vi "IV.vi"(2 "Run uninterrupted?":bool, 3 "Device Category IN:":string(combo)="Mini" caption="Device Category:", 4 "Batch No. IN:":string caption="Batch No.:", 5 "Sensor Serial No. IN:":string caption="Sensor Serial No.:", 6 "DB Serial No. IN:":string caption="DB Serial No.:") -> (0 "Done!":bool)   [LabVIEW 2019]
doc: "Performs IV measurements according to ATLAS ITk Quality Control Specifications."
uses:
  general_VIs/globals/QC_MeasurementSetup.vi
  general_VIs/globals/QC_RunInformation.vi
  InstrControl/InstrumentSetup.vi
  InstrControl/Switching/Switching.lvclass
  InstrControl/SupplyControl/SupplyControl.lvclass
  InstrControl/ArduinoControl/ArduinoControl.lvclass
  <vilib>/Analysis/NI_AALBase.lvlib
  InstrControl/InstrControl.lvclass
panel:
  out "Measurement Configuration Tab":enum32{"IV Setup", "IV Scan"}(tab)
  in  "V_breakdown limit [V]":dbl=-500.0
  in  "Set current limit?":bool
  in  "Current Limit [µA]":dbl=1000.0 min=0.0001 format="%.3f"
  in  "Measurement Configurations":bool
  in  "hold steps IN":i32=6 caption="hold steps"
  in  "Initial volts [V] IN":dbl caption="Initial volts [V]"
  in  "Final volts [V] IN":dbl=-700.0 caption="Final volts [V]"
  in  "step [V] IN":dbl=10.0 caption="step [V]" format="%.1f"
  in  "step interval [s] IN":i32=10 caption="step interval [s]"
  in  "Continue":bool
  in  "Quit":bool
  out "hold steps":i32=6
  out "RH":dbl[](array[numeric]) caption="RH [%]" format="%#.2f"
  out "Temp.":dbl[](array[numeric]) caption="Temp. [°C]" format="%#.2f"
  out "Current":dbl[](array[numeric]) caption="Current [nA]"
  out "Volts":dbl[](array[numeric]) caption="Volts [V]"
  out "step interval [s]":i32=10
  out "step [V]":dbl=10.0 format="%.1f"
  out "Final volts [V]":dbl=-700.0 format="%.1f"
  out "Initial volts [V]":dbl format="%.1f"
  out "Igraph":cluster{dbl[], dbl[]}(graph)
  in  "Scales":T1(ring)
  in  "Iscale":enum16{"nanoAmps", "microAmps", "milliAmps"}(ring)
  out "positive ramp?":bool
  out "DUT Description/Hardware Tab":enum32{"IV Setup", "IV Scan"}(tab)
  in  "Switching":string(combo)="LXIPXI Switching"
  in  "Hardware Configurations":bool
  in  "User:":string(combo)="Xavi"
  in  "IV Supply":string(combo)="Keithley 2410"
  in  "Temperature":enum16{"Read Arduino", "Enter manually"}(ring)
  in  "Manufacturer:":string(combo)="Hamamatsu"
  in  "abort":bool
  out "Device Category:":string
  out "DB Serial No.:":string
  out "Current Volts:":dbl format="%.2f"
  in  "quit (no save)":bool
  in  "Quit & Save":bool
  out "Bias On/Off:":bool
  out "STATUS 1":string
  out "Initiated:":string
  out "Sensor No.:":string
  out "No of steps":u32
  out "Current reading No.":u32
  out "Last reading at:":string
  # "University of\nCambridge"
  # "Strip Sensor QC: IV"
  # "Vertical Scale:"
  # "Measurement Configuration"
  # "IV Scan parameters:"
  # "Last 5 readings:"
  # "n-4"
  # "n-3"
  # "n-2"
  # "n-1"
  # "n"
  # "DUT Description"
  # "Hardware"
  # "DUT & Test Description:"
  # "Current status:"
  # "Rdg No:"
  # "out of"
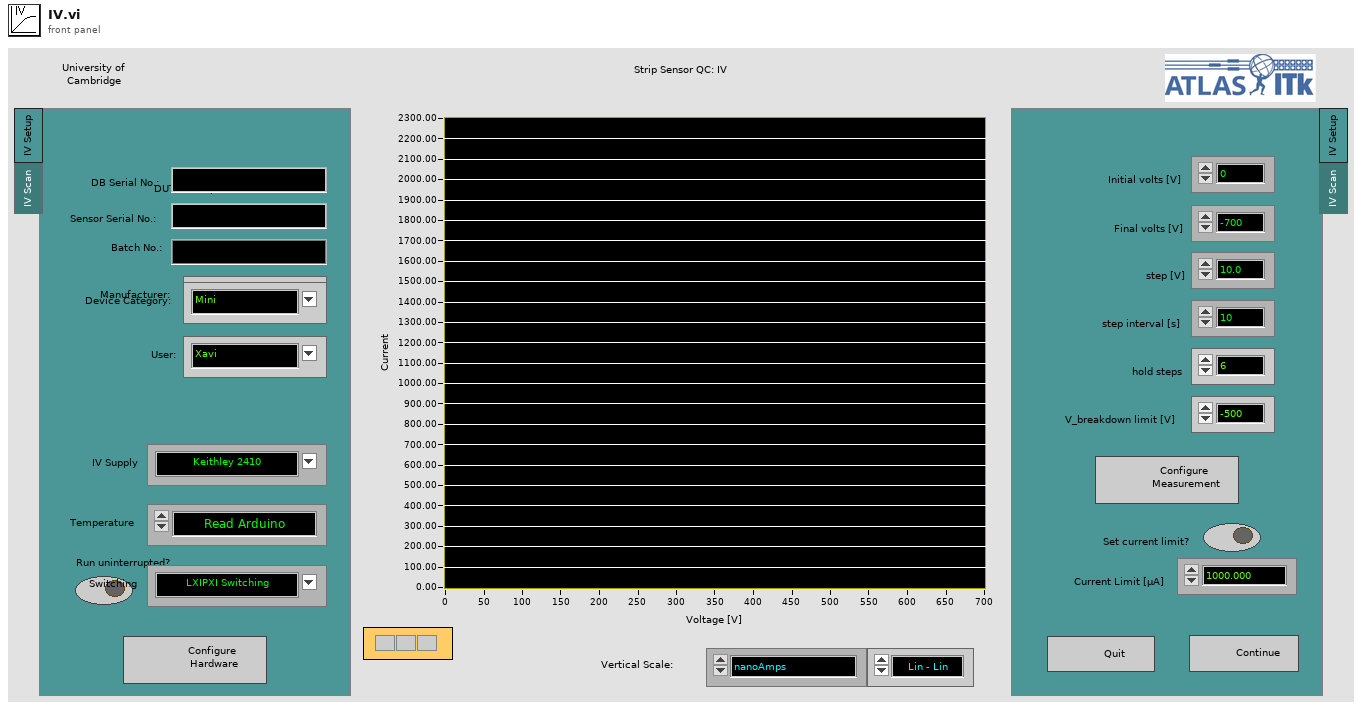
[diagram p1: front panel]
types:
  T1 = enum16{"Lin - Lin", "Log - Lin", "Lin - Log", "Log - log"}
  T2 = enum16{"Supply", "LCR", "Multimeter", "Switching"}
  T3 = enum16{"Reset", "Read Array", "Read Element", "Write Element", "Write Array", "Add Element", "Add Array"}
  T4 = enum16{"Reset", "Ground", "Striptest Bias", "Striptest SMU", "Striptest LCR", "IV", "CV", "Interstrip Cap", "Interstrip Res"}
  T5 = enum32{"IV", "CV", "Stability", "Striptest", "Cis", "Ris", "PTP"}
  T6 = cluster{"Supply":refnum<class "SupplyControl.lvclass">, "Initial Voltage [V]":dbl, "Final Voltage [V]":dbl, "Step Size [V]":dbl, "Step Interval [s]":i32, "Number Of Steps":u32, "Ramp down steps [V]":dbl, "Ramp down Interval [s]":i32, "hold steps":i32, "Set Current Limit?":bool, "Current Limit [µA]":dbl, "Temperature Readout":enum16{"Read Arduino", "Enter manually"}, "Arduino":refnum<class "ArduinoControl.lvclass">, "Supply Name":string, "V_breakdown Limit [V]":dbl, "Switching":refnum<class "Switching.lvclass">, "Matrix used?":bool, "Matrix X Channels":cluster{"Bias Supply / SMU LO":i32, "Bias Supply / SMU HI":i32, "CV Box LO":i32, "CV Box HI":i32, "CV Box LO IN":i32, "CV Box HI IN":i32, "Volt meter LO":i32, "Volt meter HI":i32, "Mux1 C1":i32, "Mux1 C2":i32, "Mux2 C1":i32, "Mux2 C2":i32}}
  T7 = cluster{"Sensor Serial No.:":string, "Wafer Serial No.:":string, "Batch:":string, "Manufacturer:":string, "Device Category:":string, "Database Serial No.:":string, "Date Initiated:":string, "Time Initiated:":string, "Test":string, "Instruments used:":string, "Probeplan used:":string, "End of Run comment:":string, "User:":string}
  T8 = cluster{"Institute":string, "Manufacturers":string[], "Devices":string[], "Serialnumbers Lookup DB":string, "Data directory":string, "Backup & screenshot directory":string, "List of known users":string[], "Measurement switch not used":bool, "Measurement Switch":string, "DUT Switch":string}
  T9 = cluster{"VISA address":refnum<visa-resource-name>, "T sensor":enum16{"SHT", "DS"}, "Arduino":refnum<class "ArduinoControl.lvclass">}
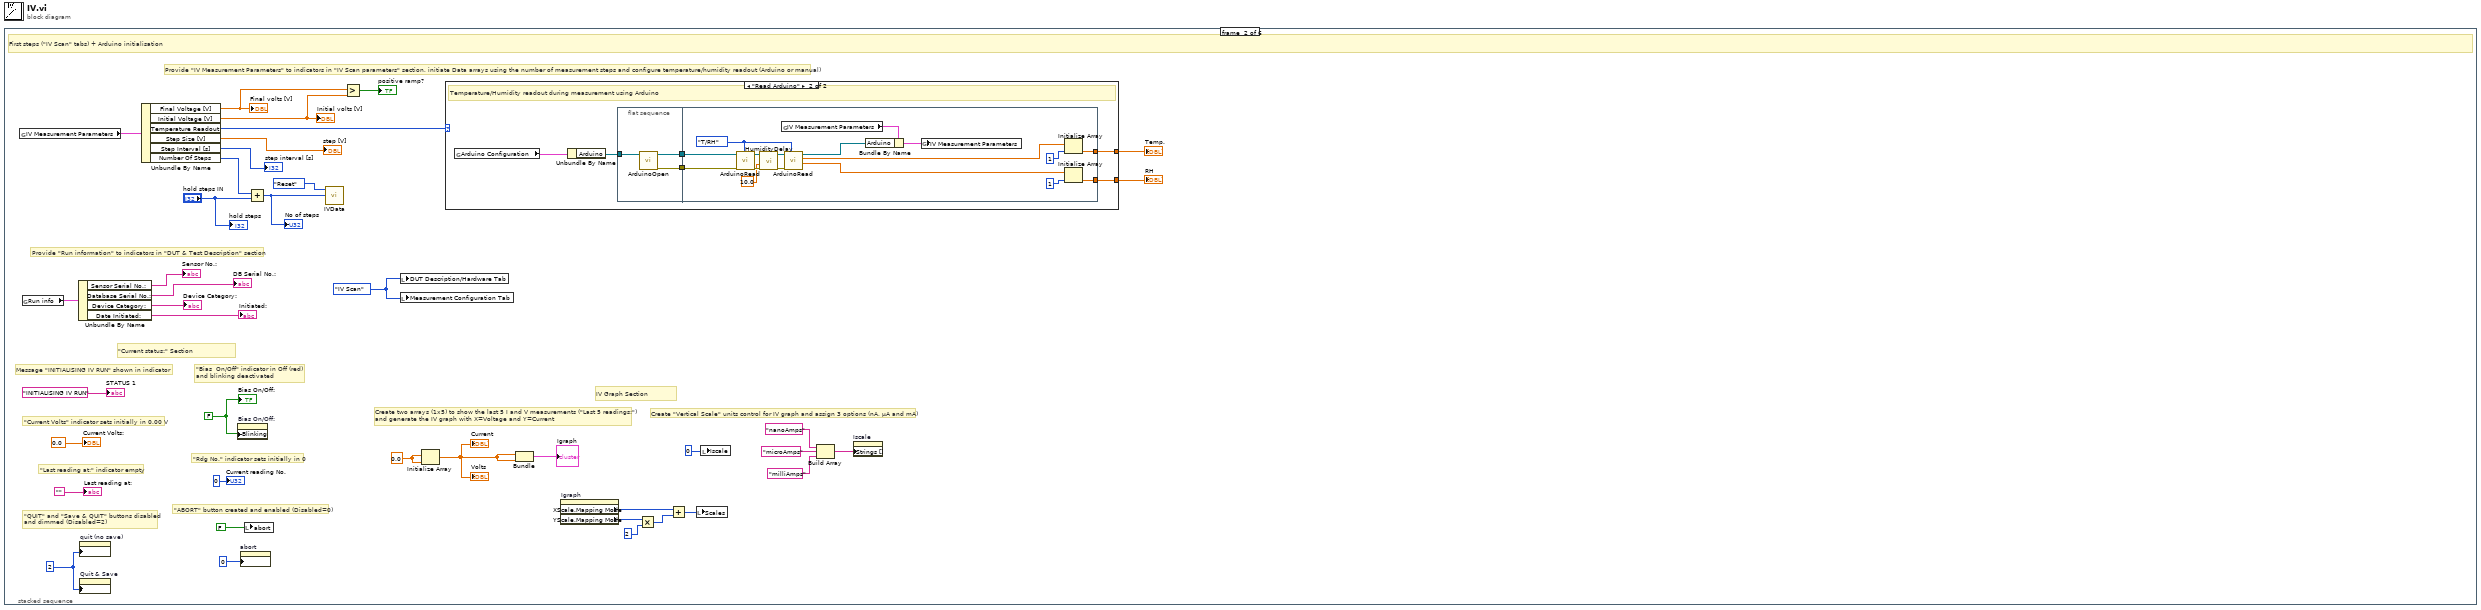
[diagram p0: block diagram]
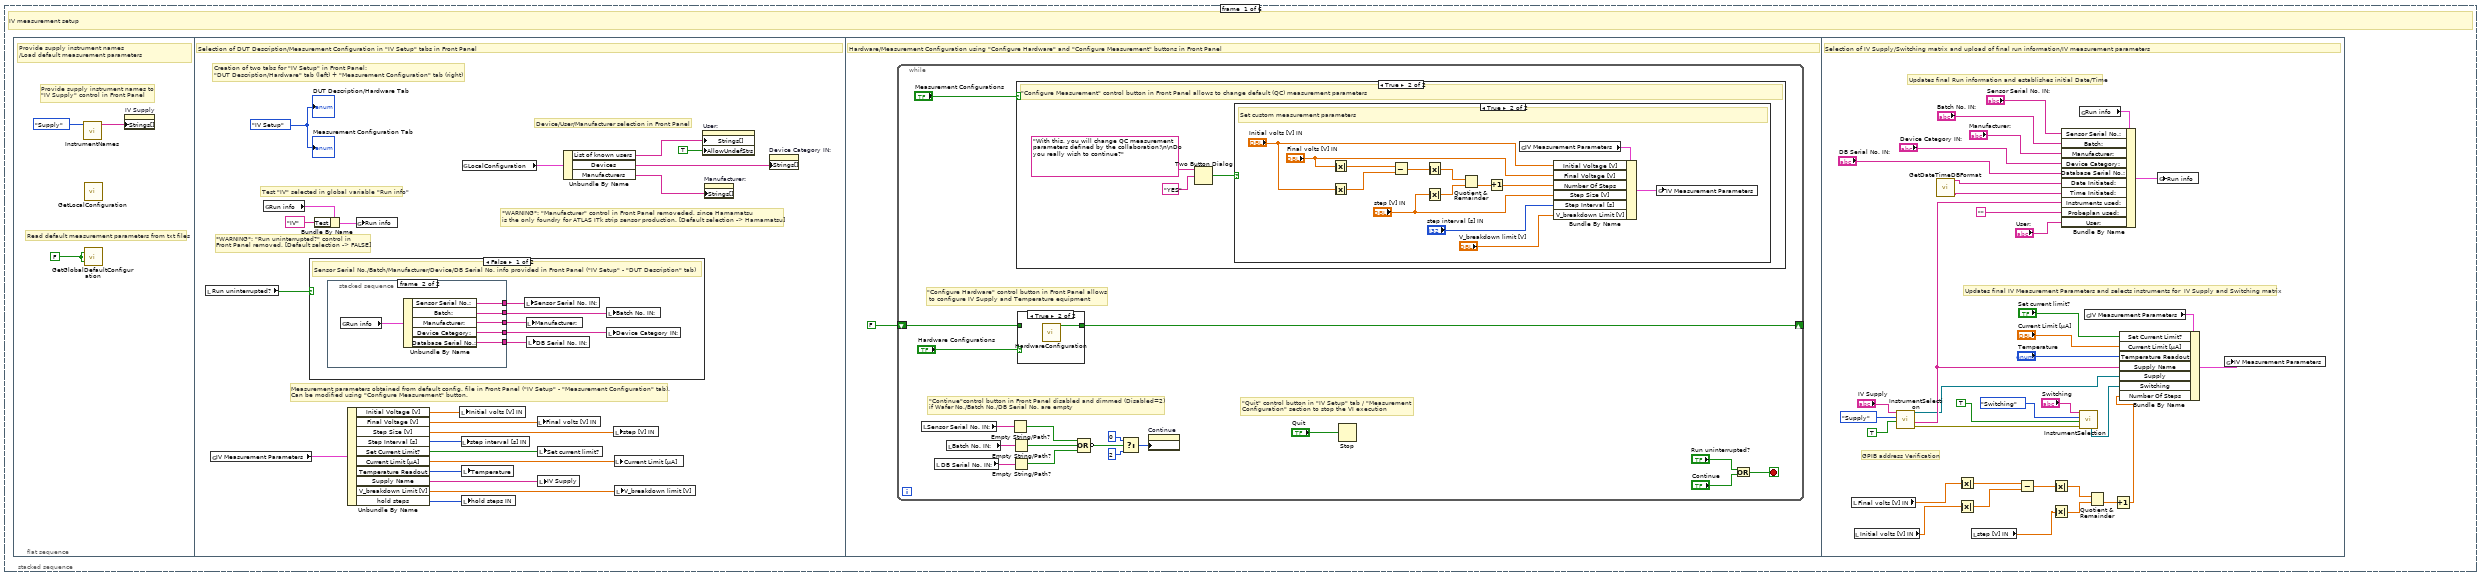
[diagram p2: hidden frame]
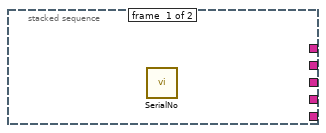
[diagram p3: hidden frame]
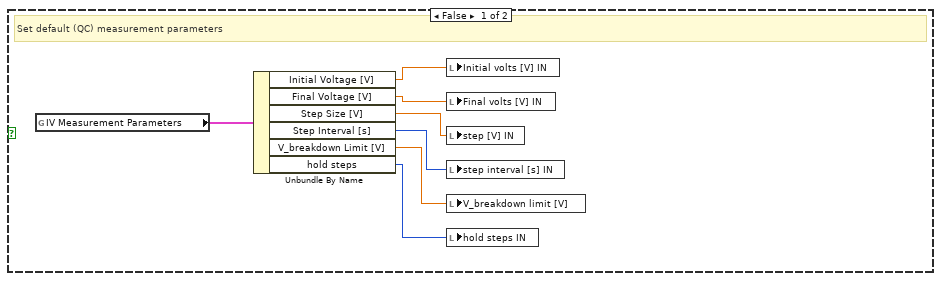
[diagram p6: hidden frame]
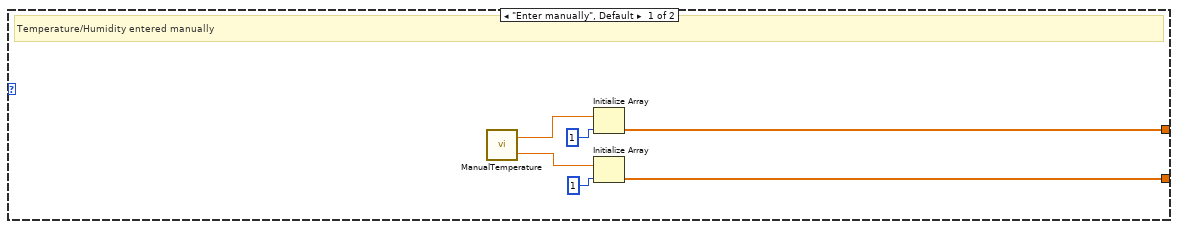
[diagram p8: hidden frame]
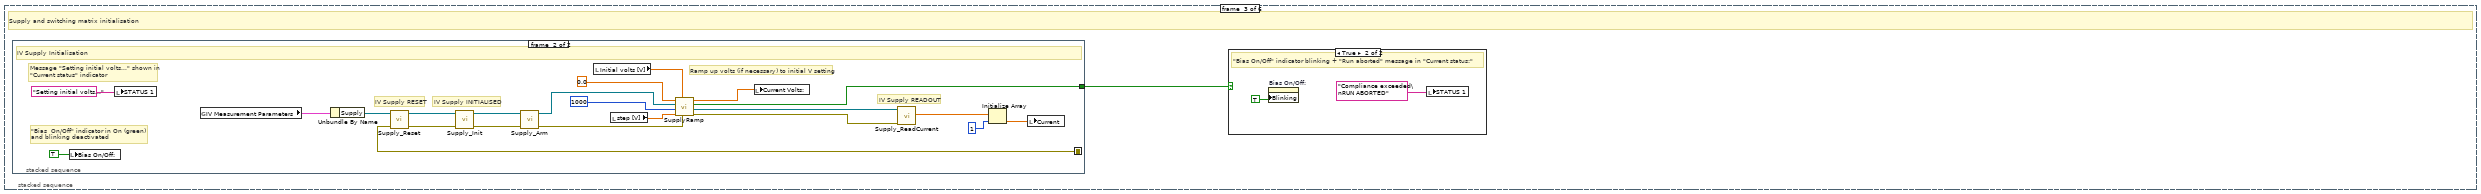
[diagram p9: hidden frame]
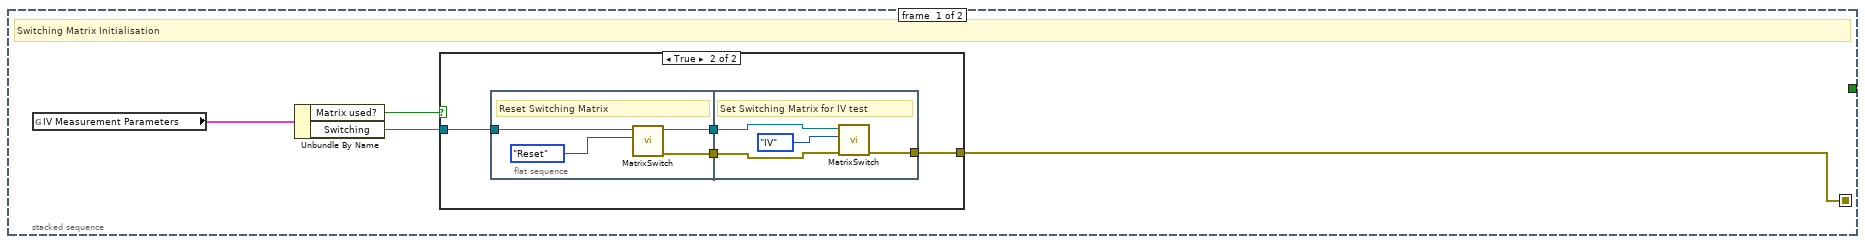
[diagram p10: hidden frame]
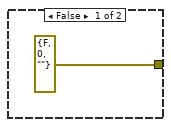
[diagram p11: hidden frame]
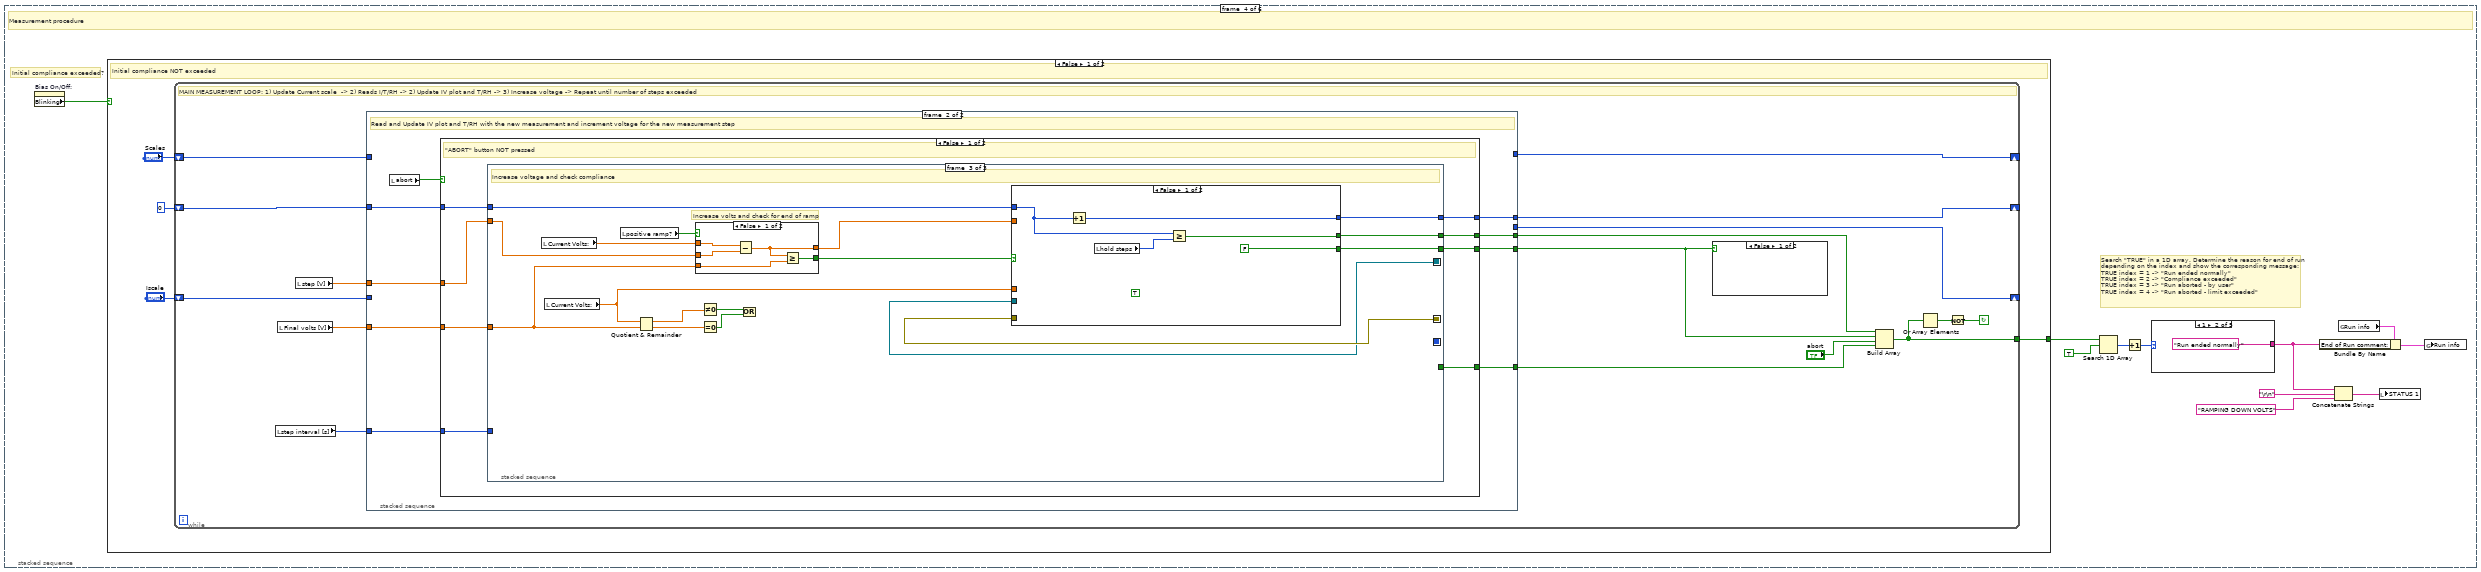
[diagram p13: hidden frame]
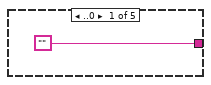
[diagram p14: hidden frame]
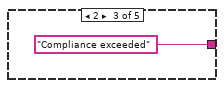
[diagram p15: hidden frame]
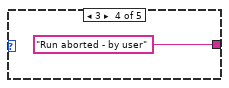
[diagram p16: hidden frame]
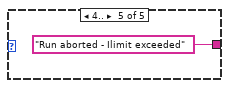
[diagram p17: hidden frame]
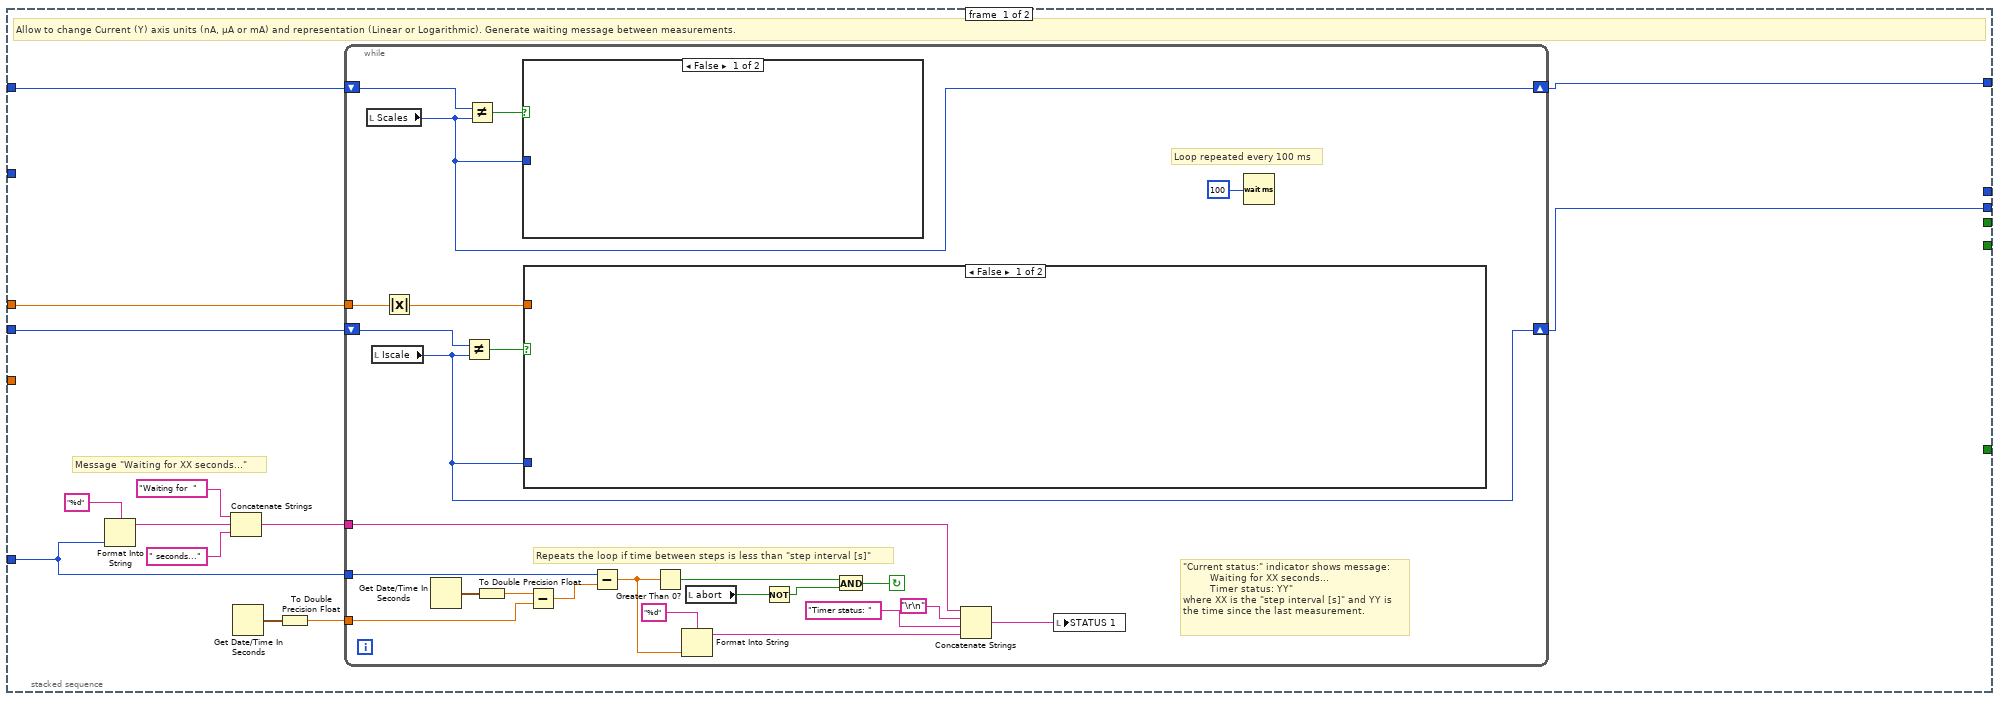
[diagram p18: hidden frame]
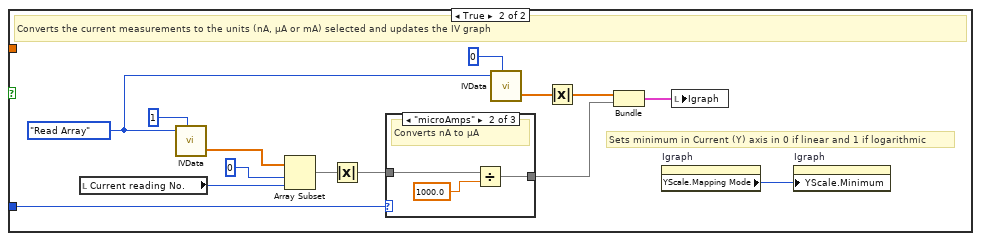
[diagram p19: hidden frame]
diagram:
  n1 = stacked-sequence {
    frame #0 {
      # "IV measurement setup"
      n2 = flat-sequence {
        frame #0 {
          w3 = FALSE
          # "Read default measurement parameters from txt files"
          # "Provide supply instrument names to \n\"IV Supply\" control in Front Panel"
          # "Provide supply instrument names\n/Load default measurement parameters"
          n3 = call "InstrumentNames.vi"("Instrument type"=T2."Supply") -> ("Instrument names"=w1:string[])  [unwired: 9 in, 1 out]
          n4 = call "GetLocalConfiguration.vi"() -> ()  [unwired: 3 in, 1 out]
          n5 = call "GetGlobalDefaultConfiguration.vi"("DO NOT override instruments"=w3, "Read defaults?"=w3) -> ()  [unwired: 1 in, 1 out]
          n6 = property on="IV Supply" class="CmbBox"("Strings[]"=w1) -> ()  [unwired: 2 in, 2 out]
        }
        frame #1 {
          w12 = enum32{"IV Setup", "IV Scan"}."IV Setup" ("Tab Control")
          # "Device/User/Manufacturer selection in Front Panel"
          # "*WARNING*: \"Manufacturer\" control in Front Panel removeded, since Hamamatsu \nis the only foundry for ATLAS ITk strip sensor production. [Default selection -> Hamamatsu]"
          # "Measurement parameters obtained from default config. file in Front Panel (\"IV Setup\" - \"Measurement Configuration\" tab).\nCan be modified using \"Configure Measurement\" button."
          # "Test \"IV\" selected in global variable \"Run info\""
          # "Creation of two tabs for \"IV Setup\" in Front Panel:\n\"DUT Description/Hardware\" tab (left) + \"Measurement Configuration\" tab (right)"
          # "*WARNING*: \"Run uninterrupted?\" control in \nFront Panel removed. [Default selection -> FALSE]"
          # "Selection of DUT Description/Measurement Configuration in \"IV Setup\" tabs in Front Panel"
          n7 = local read "Run uninterrupted?"() -> (w16:bool)
          n8 = global read "QC_MeasurementSetup.vi" "IV Measurement Parameters"() -> (w22:T6)
          n9 = global read "QC_RunInformation.vi" "Run info"() -> (w15:T7)
          n10 = case shown="False" w16 {
            frame False {
              # "Sensor Serial No./Batch/Manufacturer/Device/DB Serial No. info provided in Front Panel (\"IV Setup\" - \"DUT Description\" tab)"
              n11 = stacked-sequence {
                tunnel: [_ w35] -> w28
                tunnel: [_ w34] -> w27
                tunnel: [_ w33] -> w26
                tunnel: [_ w32] -> w29
                tunnel: [_ w30] -> w25
                frame #0 {
                  n12 = call "SerialNo.vi"() -> ()  [unwired: 5 in, 1 out]
                }
                frame #1 {
                  n13 = global read "QC_RunInformation.vi" "Run info"() -> (w31:T7)
                  n14 = Unbundle By Name(w31) -> ("Sensor Serial No.:"=w35:string, "Batch:"=w34:string, "Manufacturer:"=w33:string, "Device Category:"=w32:string, "Database Serial No.:"=w30:string)
                }
              }
              n15 = local write "Sensor Serial No. IN:"(w28) -> ()
              n16 = local write "Manufacturer:"(w26) -> ()
              n17 = local write "DB Serial No. IN:"(w25) -> ()
              n18 = local write "Batch No. IN:"(w27) -> ()
              n19 = local write "Device Category IN:"(w29) -> ()
            }
            frame True {
            }
          }
          n20 = Bundle By Name(cluster=w15, "Test"="IV") -> (w13:T7)
          n21 = Unbundle By Name(w22) -> ("Initial Voltage [V]"=w10:dbl, "Final Voltage [V]"=w9:dbl, "Step Size [V]"=w8:dbl, "Step Interval [s]"=w11:i32, "Set Current Limit?"=w21:bool, "Current Limit [µA]"=w20:dbl, "Temperature Readout"=w24:enum16{"Read Arduino", "Enter manually"}, "Supply Name"=w23:string, "V_breakdown Limit [V]"=w7:dbl, "hold steps"=w6:i32)
          n22 = global write "QC_RunInformation.vi" "Run info"(w13) -> ()
          n23 = local write "Initial volts [V] IN"(w10) -> ()
          n24 = local write "step interval [s] IN"(w11) -> ()
          n25 = local write "Temperature"(w24) -> ()
          n26 = local write "hold steps IN"(w6) -> ()
          n27 = global read "QC_RunInformation.vi" "LocalConfiguration"() -> (w19:T8)
          n28 = local write "Final volts [V] IN"(w9) -> ()
          n29 = local write "Set current limit?"(w21) -> ()
          n30 = local write "IV Supply"(w23) -> ()
          n31 = Unbundle By Name(w19) -> ("List of known users"=w18:string[], "Devices"=w5:string[], "Manufacturers"=w4:string[])
          n32 = local write "step [V] IN"(w8) -> ()
          n33 = local write "Current Limit [µA]"(w20) -> ()
          n34 = local write "V_breakdown limit [V]"(w7) -> ()
          n35 = property on="User:" class="CmbBox"("Strings[]"=w18, "AllowUndefStrs"=TRUE) -> ()  [unwired: 2 in, 2 out]
          n36 = property on="Manufacturer:" class="CmbBox"("Strings[]"=w4) -> ()  [unwired: 2 in, 2 out]
          n37 = property on="Device Category IN:" class="CmbBox"("Strings[]"=w5) -> ()  [unwired: 2 in, 2 out]
          "DUT Description/Hardware Tab" <- w12
          "Measurement Configuration Tab" <- w12
        }
        frame #2 {
          # "Hardware/Measurement Configuration using \"Configure Hardware\" and \"Configure Measurement\" buttons in Front Panel"
          n38 = while {
            shift-right: [w44] -> _
            shift-left: FALSE -> [w43]
            stop <- w40 stop-if-true
            # "\"Continue\"control button in Front Panel disabled and dimmed (Disabled=2) \nif Wafer No./Batch No./DB Serial No. are empty"
            # "\"Configure Hardware\" control button in Front Panel allows\n to configure IV Supply and Temperature equipment"
            # "\"Quit\" control button in \"IV Setup\" tab / \"Measurement \nConfiguration\" section to stop the VI execution"
            n39 = local read "Sensor Serial No. IN:"() -> (w53:string)
            n40 = local read "DB Serial No. IN:"() -> (w38:string)
            n41 = local read "Batch No. IN:"() -> (w46:string)
            n42 = Empty String/Path?(string/path=w53) -> (empty?=w52:bool)
            n43 = Empty String/Path?(string/path=w46) -> (empty?=w45:bool)
            n44 = Empty String/Path?(string/path=w38) -> (empty?=w37:bool)
            n45 = case shown="True" "Measurement Configurations" {
              frame False {
              }
              frame True {
                # "\"Configure Measurement\" control button in Front Panel allows to change default (QC) measurement parameters"
                n46 = Two Button Dialog(message="With this, you will change QC measurement parameters defined by the collaboration!\n\nDo you really wish to continue?", 2:"YES") -> (T button?=w55:bool)  [unwired: 1 in]
                n47 = case shown="True" w55 {
                  frame False {
                    # "Set default (QC) measurement parameters"
                    n48 = global read "QC_MeasurementSetup.vi" "IV Measurement Parameters"() -> (w64:T6)
                    n49 = Unbundle By Name(w64) -> ("Initial Voltage [V]"=w62:dbl, "Final Voltage [V]"=w63:dbl, "Step Size [V]"=w61:dbl, "Step Interval [s]"=w60:i32, "V_breakdown Limit [V]"=w59:dbl, "hold steps"=w58:i32)
                    n50 = local write "Initial volts [V] IN"(w62) -> ()
                    n51 = local write "Final volts [V] IN"(w63) -> ()
                    n52 = local write "step [V] IN"(w61) -> ()
                    n53 = local write "step interval [s] IN"(w60) -> ()
                    n54 = local write "V_breakdown limit [V]"(w59) -> ()
                    n55 = local write "hold steps IN"(w58) -> ()
                  }
                  frame True {
                    # "Set custom measurement parameters"
                    n56 = Absolute Value(x="Final volts [V] IN") -> (abs(x)=w76:dbl)
                    n57 = Absolute Value(x="Initial volts [V] IN") -> (abs(x)=w75:dbl)
                    n58 = Subtract(x=w76, y=w75) -> (x-y=w70:dbl)
                    n59 = Absolute Value(x=w70) -> (abs(x)=w72:dbl)
                    n60 = Absolute Value(x="step [V] IN") -> (abs(x)=w71:dbl)
                    n61 = Quotient & Remainder(x=w72, y=w71) -> (floor(x/y)=w69:dbl)  [unwired: 1 out]
                    n62 = Increment(x=w69) -> (x+1=w67:dbl)
                    n63 = global read "QC_MeasurementSetup.vi" "IV Measurement Parameters"() -> (w78:T6)
                    n64 = Bundle By Name(cluster=w78, "Initial Voltage [V]"="Initial volts [V] IN", "Final Voltage [V]"="Final volts [V] IN", "Number Of Steps"=w67, "Step Size [V]"="step [V] IN", "Step Interval [s]"="step interval [s] IN", "V_breakdown Limit [V]"="V_breakdown limit [V]") -> (w77:T6)
                    n65 = global write "QC_MeasurementSetup.vi" "IV Measurement Parameters"(w77) -> ()
                  }
                }
              }
            }
            n66 = case shown="True" "Hardware Configurations" {
              tunnel: [w79 w80] -> w44
              tunnel: w43 -> [w79 _]
              frame False {
              }
              frame True {
                n67 = call "HardwareConfiguration.vi"() -> ("configured?"=w80:bool)  [unwired: 11 in]
              }
            }
            n68 = Compound Arithmetic op=OR(w52, w45, w37) -> (invert w51:bool)
            n69 = Select(t=0, s=w51, f=2) -> (s? t:f=w48:i32)
            n70 = property on="Continue" class="Bool"("DisabledEnum"=w48) -> ()  [unwired: 2 in, 2 out]
            n71 = Stop(stop? (T)="Quit") -> ()
            n72 = Or(x="Run uninterrupted?", y="Continue") -> (x .or. y?=w40:bool)
          }
        }
        frame #3 {
          # "GPIB address Verification"
          # "Updates final IV Measurement Parameters and selects instruments for  IV Supply and Switching matrix"
          # "Updates final Run information and establishes initial Date/Time"
          # "Selection of IV Supply/Switching matrix and upload of final run information/IV measurement parameters"
          n73 = local read "Final volts [V] IN"() -> (w84:dbl)
          n74 = local read "Initial volts [V] IN"() -> (w85:dbl)
          n75 = call "InstrumentSelection.vi"("Verify GPIB address"=TRUE, "Instrument type"=T2."Supply", "Instrument name IN"="IV Supply") -> ("error out"=w101:errorcluster, "Instrument name OUT"=w104:string, "Supply"=w103:refnum<class "SupplyControl.lvclass">)  [unwired: 3 in, 3 out]
          n76 = call "GetDateTimeDBFormat.vi"() -> ("Time in 24h format, e.g. 13:40:54"=w81:string, "Abbreviated Date, e.g. 13 Nov 2020"=w82:string)  [unwired: 10 in]
          n77 = Absolute Value(x=w84) -> (abs(x)=w92:dbl)
          n78 = Absolute Value(x=w85) -> (abs(x)=w91:dbl)
          n79 = local read "step [V] IN"() -> (w86:dbl)
          n80 = Subtract(x=w92, y=w91) -> (x-y=w88:dbl)
          n81 = Absolute Value(x=w88) -> (abs(x)=w90:dbl)
          n82 = Absolute Value(x=w86) -> (abs(x)=w89:dbl)
          n83 = global read "QC_RunInformation.vi" "Run info"() -> (w112:T7)
          n84 = Bundle By Name(cluster=w112, "Sensor Serial No.:"="Sensor Serial No. IN:", "Batch:"="Batch No. IN:", "Manufacturer:"="Manufacturer:", "Device Category:"="Device Category IN:", "Database Serial No.:"="DB Serial No. IN:", "Date Initiated:"=w82, "Time Initiated:"=w81, "Instruments used:"=w104, "Probeplan used:"="", "User:"="User:") -> (w111:T7)
          n85 = call "InstrumentSelection.vi"("error in (no error)"=w101, "Verify GPIB address"=TRUE, "Instrument type"=T2."Switching", "Instrument name IN"="Switching") -> ("Switching"=w100:refnum<class "Switching.lvclass">)  [unwired: 2 in, 5 out]
          n86 = global read "QC_MeasurementSetup.vi" "IV Measurement Parameters"() -> (w115:T6)
          n87 = Quotient & Remainder(x=w90, y=w89) -> (floor(x/y)=w87:dbl)  [unwired: 1 out]
          n88 = Increment(x=w87) -> (x+1=w83:dbl)
          n89 = Bundle By Name(cluster=w115, "Set Current Limit?"="Set current limit?", "Current Limit [µA]"="Current Limit [µA]", "Temperature Readout"="Temperature", "Supply Name"=w104, "Supply"=w103, "Switching"=w100, "Number Of Steps"=w83) -> (w116:T6)
          n90 = global write "QC_RunInformation.vi" "Run info"(w111) -> ()
          n91 = global write "QC_MeasurementSetup.vi" "IV Measurement Parameters"(w116) -> ()
        }
      }
    }
    frame #1 {
      w123 = enum32{"IV Setup", "IV Scan"}."IV Scan" ("Tab Control")
      w140 = 2
      w146 = 0.0
      w139 = FALSE ("Visible")
      # "IV Graph Section"
      # "\"Current status:\" Section"
      # "Create two arrays (1x5) to show the last 5 I and V measurements (\"Last 5 readings:\") \nand generate the IV graph with X=Voltage and Y=Current"
      # "\"Bias  On/Off\" indicator in Off (red)\nand blinking deactivated"
      # "\"Rdg No.\" indicator sets initially in 0"
      # "\"ABORT\" button created and enabled (Disabled=0)"
      # "\"Current Volts\" indicator sets initially in 0.00 V"
      # "\"Last reading at:\" indicator empty"
      # "\"QUIT\" and \"Save & QUIT\" buttons disabled\nand dimmed (Disabled=2)"
      # "Message \"INITIALISING IV RUN\" shown in indicator"
      # "Create \"Vertical Scale\" units control for IV graph and assign 3 options (nA, µA and mA)"
      # "Provide \"Run information\" to indicators in \"DUT & Test Description\" section"
      # "Provide \"IV Measurement Parameters\" to indicators in \"IV Scan parameters\" section, initiate Data arrays using the number of measurement steps and configure temperature/humidity readout (Arduino or manual)"
      # "First steps (\"IV Scan\" tabs) + Arduino initialisation"
      n92 = global read "QC_MeasurementSetup.vi" "IV Measurement Parameters"() -> (w130:T6)
      n93 = global read "QC_RunInformation.vi" "Run info"() -> (w155:T7)
      n94 = Unbundle By Name(w155) -> ("Sensor Serial No.:"=→"Sensor No.:":string, "Database Serial No.:"=→"DB Serial No.:":string, "Device Category:"=→"Device Category:":string, "Date Initiated:"=→"Initiated:":string)
      n95 = property on="quit (no save)" class="Bool"("DisabledEnum"=w140) -> ()  [unwired: 2 in, 2 out]
      n96 = property on="Quit & Save" class="Bool"("DisabledEnum"=w140) -> ()  [unwired: 2 in, 2 out]
      n97 = Unbundle By Name(w130) -> ("Final Voltage [V]"=w118:dbl, "Initial Voltage [V]"=w119:dbl, "Temperature Readout"=w120:enum16{"Read Arduino", "Enter manually"}, "Step Size [V]"=→"step [V]":dbl, "Step Interval [s]"=→"step interval [s]":i32, "Number Of Steps"=w121:u32)
      "Initial volts [V]" <- w119
      "Final volts [V]" <- w118
      n98 = property on="Bias On/Off:" class="Bool (strict)"("Blinking"=w139) -> ()  [unwired: 2 in, 2 out]
      n99 = property on="abort" class="Bool (strict)"("DisabledEnum"=0) -> ()  [unwired: 2 in, 2 out]
      n100 = local write "abort"(FALSE) -> ()
      n101 = Add(x=w121, y="hold steps IN") -> (x+y=w126:u32)
      "No of steps" <- w126
      n102 = call "IVData.vi"("Action"=T3."Reset", "Array Size / Index"=w126) -> ()  [unwired: 3 in, 2 out]
      n103 = Greater?(x=w118, y=w119) -> (0:→"positive ramp?":bool)
      n104 = local write "DUT Description/Hardware Tab"(w123) -> ()
      n105 = local write "Measurement Configuration Tab"(w123) -> ()
      n106 = Initialize Array(w146, w146) -> (w125:dbl[])
      "Volts" <- w125
      "Current" <- w125
      n107 = case shown="\"Read Arduino\"" w120 {
        tunnel: [w161 w168] -> w143
        tunnel: [w158 w167] -> w131
        frame "Enter manually", Default {
          # "Temperature/Humidity entered manually"
          n108 = call "ManualTemperature.vi"() -> ("Humidity [%] out"=w157:dbl, "Temperature [°C] out"=w162:dbl)
          n109 = Initialize Array(w162, 1) -> (w161:dbl[])
          n110 = Initialize Array(w157, 1) -> (w158:dbl[])
        }
        frame "Read Arduino" {
          # "Temperature/Humidity readout during measurement using Arduino"
          n111 = global read "InstrumentSetup.vi" "Arduino Configuration"() -> (w164:T9)
          n112 = Unbundle By Name(w164) -> ("Arduino"=w163:refnum<class "ArduinoControl.lvclass">)
          n113 = flat-sequence {
            tunnel: [w169] -> w166
            tunnel: [w171] -> w165
            tunnel: w163 -> [w170]
            tunnel: [w188] -> w168
            tunnel: [w185] -> w167
            tunnel: w166 -> [w179]
            tunnel: w165 -> [w178]
            frame #0 {
              n114 = call "ArduinoOpen.vi"("ArduinoControl in"=w170) -> ("error out"=w171:errorcluster, "ArduinoControl out"=w169:refnum<class "ArduinoControl.lvclass">)  [unwired: 9 in]
            }
            frame #1 {
              w177 = enum16{"T/RH", "Interlock", "Edgesense"}."T/RH" ("Arduino function")
              n115 = call "ArduinoRead.vi"("Arduino function"=w177, "error in (no error)"=w178, "ArduinoControl in"=w179) -> ("error out"=w173:errorcluster, "ArduinoControl out"=w174:refnum<class "ArduinoControl.lvclass">)  [unwired: 3 in, 4 out]
              n116 = call "HumidityDelay.vi"("error in (no error)"=w173, "Start Humidity"=10.0, "ArduinoControl in"=w174) -> ("error out"=w176:errorcluster, "ArduinoControl out"=w175:refnum<class "ArduinoControl.lvclass">)  [unwired: 7 in]
              n117 = global read "QC_MeasurementSetup.vi" "IV Measurement Parameters"() -> (w181:T6)
              n118 = call "ArduinoRead.vi"("Arduino function"=w177, "error in (no error)"=w176, "ArduinoControl in"=w175) -> ("rel. Humidity [%]"=w183:dbl, "Temperature [°C]"=w184:dbl, "ArduinoControl out"=w182:refnum<class "ArduinoControl.lvclass">)  [unwired: 3 in, 3 out]
              n119 = Bundle By Name(cluster=w181, "Arduino"=w182) -> (w180:T6)
              n120 = global write "QC_MeasurementSetup.vi" "IV Measurement Parameters"(w180) -> ()
              n121 = Initialize Array(w184, 1) -> (w188:dbl[])
              n122 = Initialize Array(w183, 1) -> (w185:dbl[])
            }
          }
        }
      }
      "Temp." <- w143
      "RH" <- w131
      n123 = Bundle(w125, w125) -> (→"Igraph":cluster{dbl[], dbl[]})  [unwired: 1 in]
      n124 = property on="Igraph" class="XYGraph (strict)"() -> ("XScale.Mapping Mode"=w134:u8, "YScale.Mapping Mode"=w133:u8)  [unwired: 2 in, 2 out]
      n125 = Multiply(x=w133, y=2) -> (x*y=w136:i32)
      n126 = Add(x=w134, y=w136) -> (x+y=w132:i32)
      n127 = local write "Scales"(w132) -> ()
      n128 = local write "Iscale"(u16 0 ("Scale")) -> ()
      n129 = Build Array("nanoAmps", "microAmps", "milliAmps") -> (w152:string[])
      n130 = property on="Iscale" class="Enum (strict)"("Strings []"=w152) -> ()  [unwired: 2 in, 2 out]
      "STATUS 1" <- "INITIALISING IV RUN"
      "Bias On/Off:" <- w139
      "Last reading at:" <- ""
      "Current reading No." <- u32 0 ("Current reading No.")
      "Current Volts:" <- 0.0 ("Current Volts:")
      "hold steps" <- "hold steps IN"
    }
    frame #2 {
      # "Supply and switching matrix initialisation"
      n131 = stacked-sequence {
        seq-local: [w191 _] -> [_ w207]
        tunnel: [_ w208] -> w189
        frame #0 {
          # "Switching Matrix Initialisation"
          n132 = global read "QC_MeasurementSetup.vi" "IV Measurement Parameters"() -> (w190:T6)
          n133 = Unbundle By Name(w190) -> ("Matrix used?"=w193:bool, "Switching"=w192:refnum<class "Switching.lvclass">)
          n134 = case shown="True" w193 {
            tunnel: w192 -> [_ w195]
            tunnel: [errorcluster {"status"=FALSE, "code"=0, "source"=""} ("error constant") w196] -> w191
            frame False {
            }
            frame True {
              n135 = flat-sequence {
                tunnel: [w202] -> w198
                tunnel: [w201] -> w197
                tunnel: w195 -> [w200]
                tunnel: w198 -> [w206]
                tunnel: w197 -> [w205]
                tunnel: [w204] -> w196
                frame #0 {
                  # "Reset Switching Matrix"
                  n136 = call-dynamic "MatrixSwitch.vi"("Action"=T4."Reset", "Switching in"=w200) -> ("error out"=w202:errorcluster, "Switching out"=w201:refnum<class "Switching.lvclass">)  [unwired: 7 in, 1 out]
                }
                frame #1 {
                  # "Set Switching Matrix for IV test"
                  n137 = call-dynamic "MatrixSwitch.vi"("error in (no error)"=w206, "Action"=T4."IV", "Switching in"=w205) -> ("error out"=w204:errorcluster)  [unwired: 6 in, 2 out]
                }
              }
            }
          }
        }
        frame #1 {
          # "IV Supply READOUT"
          # "IV Supply INITIALISED"
          # "IV Supply RESET"
          # "Message \"Setting initial volts...\" shown in \n\"Current status\" indicator"
          # "\"Bias  On/Off\" indicator in On (green)\nand blinking deactivated"
          # "Ramp up volts (if necessary) to initial V setting"
          # "IV Supply Initialisation"
          n138 = local write "Bias On/Off:"(TRUE ("Compliance?")) -> ()
          n139 = local write "STATUS 1"("Setting initial volts..." ("STATUS 1")) -> ()
          n140 = global read "QC_MeasurementSetup.vi" "IV Measurement Parameters"() -> (w224:T6)
          n141 = Unbundle By Name(w224) -> ("Supply"=w221:refnum<class "SupplyControl.lvclass">)
          n142 = call-dynamic "Supply_Reset.vi"("error in (no error)"=w207, "SupplyControl in"=w221) -> ("error out"=w226:errorcluster, "SupplyControl out"=w228:refnum<class "SupplyControl.lvclass">)  [unwired: 8 in]
          n143 = call-dynamic "Supply_Init.vi"("error in (no error)"=w226, "SupplyControl in"=w228) -> ("error out"=w225:errorcluster, "SupplyControl out"=w227:refnum<class "SupplyControl.lvclass">)  [unwired: 8 in]
          n144 = call-dynamic "Supply_Arm.vi"("error in (no error)"=w225, "SupplyControl in"=w227) -> ("error out"=w214:errorcluster, "SupplyControl out"=w215:refnum<class "SupplyControl.lvclass">)  [unwired: 8 in]
          n145 = local read "Initial volts [V]"() -> (w216:dbl)
          n146 = local read "step [V]"() -> (w217:dbl)
          n147 = call "SupplyRamp.vi"("error in"=w214, "Requested Voltage"=w216, "Step Size"=w217, "Step Delay"=1000, "Supply IN"=w215, "Starting Voltage"=0.0) -> ("error out"=w209:errorcluster, "Supply OUT"=w210:refnum<class "SupplyControl.lvclass">, "Compliance exceeded"=w208:bool, "Current Voltage"=w220:dbl)  [unwired: 2 in]
          n148 = local write "Current Volts:"(w220) -> ()
          n149 = call-dynamic "Supply_ReadCurrent.vi"("error in (no error)"=w209, "SupplyControl in"=w210) -> ("Current in nA"=w212:dbl)  [unwired: 7 in, 2 out]
          n150 = Initialize Array(w212, 1) -> (w211:dbl[])
          n151 = local write "Current"(w211) -> ()
        }
      }
      n152 = case shown="True" w189 {
        frame False {
        }
        frame True {
          # "\"Bias On/Off\" indicator blinking + \"Run aborted\" message in \"Current status:\""
          n153 = property on="Bias On/Off:" class="Bool (strict)"("Blinking"=TRUE) -> ()  [unwired: 2 in, 2 out]
          n154 = local write "STATUS 1"("Compliance exceeded\nRUN ABORTED") -> ()
        }
      }
    }
    frame #3 {
      # "Search \"TRUE\" in a 1D array. Determine the reason for end of run \ndepending on the index and show the corresponding message:\nTRUE index = 1 -> \"Run ended normally\"\nTRUE index = 2 -> \"Compliance exceeded\"\nTRUE index = 3 -> \"Run aborted - by user\"\nTRUE index = 4 -> \"Run aborted - limit exceeded\""
      # "Initial compliance exceeded?"
      # "Measurement procedure"
      n155 = property on="Bias On/Off:" class="Bool (strict)"() -> ("Blinking"=w241:bool)  [unwired: 2 in, 2 out]
      n156 = case shown="False" w241 {
        tunnel: [w250 w508] -> w240
        frame False {
          # "Initial compliance NOT exceeded"
          n157 = while {
            shift-left: "Iscale" -> [w262]
            shift-right: [w261] -> _
            shift-left: "Scales" -> [w263]
            shift-right: [w264] -> _
            tunnel: [w260] -> w250
            shift-right: [w252] -> _
            shift-left: 0 -> [w253]
            stop <- w265 continue-if-true
            # "MAIN MEASUREMENT LOOP: 1) Update Current scale  -> 2) Reads I/T/RH -> 2) Update IV plot and T/RH -> 3) Increase voltage -> Repeat until number of steps exceeded"
            n158 = local read "step interval [s]"() -> (w257:i32)
            n159 = local read "Final volts [V]"() -> (w258:dbl)
            n160 = local read "step [V]"() -> (w259:dbl)
            n161 = stacked-sequence {
              tunnel: [w279 _] -> w264
              tunnel: w259 -> [w276 w343]
              tunnel: [_ w342] -> w255
              tunnel: w258 -> [_ w341]
              tunnel: w257 -> [w267 w340]
              tunnel: [_ w339] -> w256
              tunnel: w263 -> [w278 _]
              tunnel: w262 -> [w277 _]
              tunnel: [w275 _] -> w261
              tunnel: [_ w337] -> w251
              tunnel: w253 -> [_ w336]
              tunnel: [_ w335] -> w252
              frame #0 {
                # "Message \"Waiting for XX seconds...\""
                # "Allow to change Current (Y) axis units (nA, µA or mA) and representation (Linear or Logarithmic). Generate waiting message between measurements."
                n162 = Format Into String(format string="%d", w267) -> (resulting string=w272:string)  [unwired: 2 in, 1 out]
                n163 = Concatenate Strings("Waiting for  ", w272, " seconds...") -> (w268:string)
                n164 = Get Date/Time In Seconds() -> (seconds since 1Jan1904=w269:timestamp)
                n165 = To Double Precision Float(number=w269) -> (double precision float=w270:dbl)
                n166 = while {
                  tunnel: w276 -> [w288]
                  shift-left: w277 -> [w292]
                  shift-right: [w285] -> w275
                  shift-left: w278 -> [w293]
                  shift-right: [w294] -> w279
                  tunnel: w268 -> [w286]
                  tunnel: w267 -> [w298]
                  tunnel: w270 -> [w299]
                  stop <- w300 continue-if-true
                  # "\"Current status:\" indicator shows message:\n         Waiting for XX seconds...\n         Timer status: YY\"\nwhere XX is the \"step interval [s]\" and YY is\nthe time since the last measurement."
                  # "Repeats the loop if time between steps is less than \"step interval [s]\""
                  # "Loop repeated every 100 ms"
                  n167 = local read "Scales"() -> (w294:T1)
                  n168 = local read "Iscale"() -> (w285:enum16{"nanoAmps", "microAmps", "milliAmps"})
                  n169 = Absolute Value(x=w288) -> (abs(x)=w287:dbl)
                  n170 = Get Date/Time In Seconds() -> (seconds since 1Jan1904=w284:timestamp)
                  n171 = Not Equal?(x=w292, y=w285) -> (x != y?=w283:bool)
                  n172 = Not Equal?(x=w293, y=w294) -> (x != y?=w295:bool)
                  n173 = To Double Precision Float(number=w284) -> (double precision float=w304:dbl)
                  n174 = case shown="False" w295 {
                    tunnel: w294 -> [_ w328]
                    frame False {
                    }
                    frame True {
                      # "Linear (0) or Logarithmical (1) representation of X and Y axis in IV graph"
                      n175 = case shown="\"Log - Lin\"" w328 {
                        tunnel: [w329 1 0 w334] -> w327
                        tunnel: [w329 0 1 w334] -> w326
                        frame .."Lin - Lin" {
                          w329 = 0
                        }
                        frame "Log - Lin" {
                        }
                        frame "Lin - Log" {
                        }
                        frame "Log - log".. {
                          w334 = 1
                        }
                      }
                      n176 = property on="Igraph" class="XYGraph (strict)"("X Scale.Mapping Mode"=w327) -> ()  [unwired: 2 in, 2 out]
                      n177 = property on="Igraph" class="XYGraph (strict)"("Y Scale.Mapping Mode"=w326, "YScale.Minimum"=w326) -> ()  [unwired: 2 in, 2 out]
                    }
                  }
                  n178 = case shown="False" w283 {
                    tunnel: w287 -> [_ _]
                    tunnel: w285 -> [_ w313]
                    frame False {
                    }
                    frame True {
                      w307 = T3."Read Array" ("Action")
                      # "Sets minimum in Current (Y) axis in 0 if linear and 1 if logarithmic"
                      # "Converts the current measurements to the units (nA, µA or mA) selected and updates the IV graph"
                      n179 = local read "Current reading No."() -> (w315:u32)
                      n180 = call "IVData.vi"("Action"=w307, "Array No."=u32 1 ("Action")) -> ("Array OUT"=w316:dbl[])  [unwired: 3 in, 1 out]
                      n181 = Array Subset(array=w316, index=0, length=w315) -> (w312:dbl[])
                      n182 = Absolute Value(x=w312) -> (abs(x)=w311:dbl[])
                      n183 = case shown="\"microAmps\"" w313 {
                        tunnel: [w319 w320 w324] -> w318
                        tunnel: w311 -> [w319 w322 w325]
                        frame .."nanoAmps" {
                        }
                        frame "microAmps" {
                          # "Converts nA to µA"
                          n184 = Divide(x=w322, y=1000.0) -> (x/y=w320:dbl[])
                        }
                        frame "milliAmps".. {
                          # "Converts nA to mA"
                          n185 = Divide(x=w325, y=1000000.0) -> (x/y=w324:dbl[])
                        }
                      }
                      n186 = call "IVData.vi"("Action"=w307, "Array No."=u32 0 ("Action")) -> ("Array OUT"=w306:dbl[])  [unwired: 3 in, 1 out]
                      n187 = Absolute Value(x=w306) -> (abs(x)=w305:dbl[])
                      n188 = Bundle(w305, w318) -> (w314:cluster{dbl[], dbl[]})  [unwired: 1 in]
                      n189 = property on="Igraph" class="XYGraph (strict)"() -> ("YScale.Mapping Mode"=w309:u8)  [unwired: 2 in, 2 out]
                      n190 = local write "Igraph"(w314) -> ()
                      n191 = property on="Igraph" class="XYGraph (strict)"("YScale.Minimum"=w309) -> ()  [unwired: 2 in, 2 out]
                    }
                  }
                  n192 = Subtract(x=w304, y=w299) -> (x-y=w281:dbl)
                  n193 = Subtract(x=w298, y=w281) -> (x-y=w280:dbl)
                  n194 = Greater Than 0?(x=w280) -> (x > 0?=w282:bool)
                  n195 = Format Into String(format string="%d", w280) -> (resulting string=w302:string)  [unwired: 2 in, 1 out]
                  n196 = local read "abort"() -> (w297:bool)
                  n197 = Not(x=w297) -> (.not. x?=w303:bool)
                  n198 = And(x=w282, y=w303) -> (x .and. y?=w300:bool)
                  n199 = Concatenate Strings(w286, "\r\n", "Timer status: ", w302) -> (w296:string)
                  n200 = local write "STATUS 1"(w296) -> ()
                  n201 = Wait (ms)(milliseconds to wait=u32 100) -> ()  [unwired: 1 out]
                }
              }
              frame #1 {
                # "Read and Update IV plot and T/RH with the new measurement and increment voltage for the new measurement step"
                n202 = local read "abort"() -> (w338:bool)
                n203 = case shown="False" w338 {
                  tunnel: [w351 w505] -> w339
                  tunnel: w340 -> [w350 _]
                  tunnel: w341 -> [w349 _]
                  tunnel: [w347 w505] -> w342
                  tunnel: w343 -> [w348 _]
                  tunnel: [w346 w505] -> w337
                  tunnel: w336 -> [w345 w504]
                  tunnel: [w344 w504] -> w335
                  frame False {
                    # "\"ABORT\" button NOT pressed"
                    n204 = stacked-sequence {
                      seq-local: [w353 _ _] -> [_ w408 _]
                      seq-local: [w371 _ _] -> [_ _ w469]
                      seq-local: [w370 _ _] -> [_ _ w470]
                      tunnel: w348 -> [_ w405 w475]
                      tunnel: w349 -> [_ _ w467]
                      tunnel: [_ _ w473] -> w351
                      tunnel: [_ _ w472] -> w347
                      tunnel: w350 -> [_ _ _]
                      tunnel: [w377 _ _] -> w346
                      tunnel: w345 -> [_ w406 w461]
                      tunnel: [_ _ w460] -> w344
                      frame #0 {
                        # "Write Relative Humidity [%] in 4th column"
                        # "Write Temperature [ºC] in 3rd column"
                        # "Write Current [nA] in 2nd column"
                        # "Write Voltage [V] in 1st column"
                        # "Increase in 1 the measurement number"
                        # "Convert to nA"
                        # "Show \"Reading current ...\" message \nin \"Current status:\" indicator"
                        # "Show date/time of last measurement \nin \"Last reading at:\" indicator"
                        # "READ and WRITE Voltage/Current/Temperature/Relative Humidity. Check compliance. Show date/time of last measurement and \"Reading current...\" message."
                        n205 = global read "QC_MeasurementSetup.vi" "IV Measurement Parameters"() -> (w369:T6)
                        n206 = Get Date/Time String(want seconds? (F)=TRUE) -> (time string=w374:string)  [unwired: 2 in, 1 out]
                        n207 = local write "Last reading at:"(w374) -> ()
                        n208 = local write "STATUS 1"("Reading current ..." ("status")) -> ()
                        n209 = Unbundle By Name(w369) -> ("Supply"=w364:refnum<class "SupplyControl.lvclass">, "Set Current Limit?"=w368:bool, "Current Limit [µA]"=w366:dbl, "Arduino"=w362:refnum<class "ArduinoControl.lvclass">, "Temperature Readout"=w363:enum16{"Read Arduino", "Enter manually"})
                        n210 = call-dynamic "Supply_ReadCurrent.vi"("SupplyControl in"=w364) -> ("error out"=w370:errorcluster, "Current in nA"=w378:dbl, "SupplyControl out"=w371:refnum<class "SupplyControl.lvclass">)  [unwired: 8 in]
                        n211 = Multiply(x=w366, y=1000.0) -> (x*y=w365:dbl)
                        n212 = case shown="True" w368 {
                          tunnel: w378 -> [_ w398]
                          tunnel: w365 -> [_ w396]
                          tunnel: [FALSE w395] -> w377
                          frame False {
                            # "Measurement without compliance"
                          }
                          frame True {
                            # "Current > Compliance?"
                            n213 = Absolute Value(x=w398) -> (abs(x)=w397:dbl)
                            n214 = Greater?(x=w397, y=w396) -> (0:w395:bool)
                          }
                        }
                        n215 = case shown="\"Read Arduino\"" w363 {
                          tunnel: [w387 w393] -> w375
                          tunnel: [w384 w392] -> w372
                          tunnel: w362 -> [_ w391]
                          frame "Enter manually", Default {
                            # "Read T/RH entered manually"
                            n216 = local read "Temp."() -> (w389:dbl[])
                            n217 = local read "RH"() -> (w385:dbl[])
                            n218 = Index Array(array=w389, index=0) -> (element=w387:dbl)
                            n219 = Index Array(array=w385, index=0) -> (element=w384:dbl)
                          }
                          frame "Read Arduino" {
                            # "Read  T/RH from Arduino"
                            n220 = call "ArduinoRead.vi"("Arduino function"=enum16{"T/RH", "Interlock", "Edgesense"}."T/RH", "ArduinoControl in"=w391) -> ("rel. Humidity [%]"=w392:dbl, "Temperature [°C]"=w393:dbl)  [unwired: 4 in, 4 out]
                          }
                        }
                        n221 = local read "Current reading No."() -> (w358:u32)
                        n222 = local read "Current reading No."() -> (w352:u32)
                        n223 = local read "Current reading No."() -> (w360:u32)
                        n224 = local read "Current reading No."() -> (w359:u32)
                        n225 = local read "Current Volts:"() -> (w379:dbl)
                        n226 = local read "Current reading No."() -> (w354:u32)
                        n227 = call "IVData.vi"("Action"=T3."Write Element", "Array No."=u32 2, "Array Size / Index"=w358, "Data IN"=w375) -> ()  [unwired: 1 in, 2 out]
                        n228 = call "IVData.vi"("Action"=T3."Write Element", "Array No."=u32 3, "Array Size / Index"=w352, "Data IN"=w372) -> ()  [unwired: 1 in, 2 out]
                        n229 = call "IVData.vi"("Action"=T3."Write Element", "Array No."=0, "Array Size / Index"=w360, "Data IN"=w379) -> ()  [unwired: 1 in, 2 out]
                        n230 = call "IVData.vi"("Action"=T3."Write Element", "Array No."=u32 1, "Array Size / Index"=w359, "Data IN"=w378) -> ()  [unwired: 1 in, 2 out]
                        n231 = Increment(x=w354) -> (x+1=w353:u32)
                        n232 = local write "Current reading No."(w353) -> ()
                      }
                      frame #1 {
                        w401 = T3."Read Array" ("Action")
                        w418 = u32 5 ("y")
                        # "Update Current/Voltage plots"
                        # "Set minimum in Current (Y) axis in 0 if linear and 1 if logarithmic"
                        # "Update IV plot and show Temperature/Relative Humidity and last 5 readings of Current/Voltage"
                        n233 = Greater Than 0?(x=w406) -> (x > 0?=w407:bool)
                        n234 = Select(t=0.01, s=w407, f=w405) -> (s? t:f=w404:dbl)
                        n235 = call "IVData.vi"("Action"=w401, "Array No."=0) -> ("Array OUT"=w400:dbl[])  [unwired: 3 in, 1 out]
                        n236 = call "IVData.vi"("Action"=w401, "Array No."=1) -> ("Array OUT"=w420:dbl[])  [unwired: 3 in, 1 out]
                        n237 = Absolute Value(x=w404) -> ()  [unwired: 1 out]
                        n238 = Absolute Value(x=w400) -> (abs(x)=w399:dbl[])
                        n239 = Array Subset(array=w420, index=0, length=w408) -> (w413:dbl[])
                        n240 = Greater?(x=w408, y=w418) -> (0:w417:bool)
                        n241 = local read "Iscale"() -> (w419:enum16{"nanoAmps", "microAmps", "milliAmps"})
                        n242 = Absolute Value(x=w413) -> (abs(x)=w412:dbl[])
                        n243 = case shown="False" w417 {
                          tunnel: w408 -> [w424 w427]
                          tunnel: w418 -> [_ w426]
                          tunnel: [w424 w426] -> w416
                          tunnel: [0 w425] -> w414
                          frame False {
                          }
                          frame True {
                            n244 = Subtract(x=w427, y=w426) -> (x-y=w425:u32)
                          }
                        }
                        n245 = property on="Igraph" class="XYGraph (strict)"() -> ("YScale.Mapping Mode"=w409:u8)  [unwired: 2 in, 2 out]
                        n246 = case shown="..\"nanoAmps\"" w419 {
                          tunnel: [w452 w453 w456] -> w422
                          tunnel: w412 -> [w452 w455 w458]
                          frame .."nanoAmps" {
                          }
                          frame "microAmps" {
                            # "Converts nA to µA"
                            n247 = Divide(x=w455, y=1000.0) -> (x/y=w453:dbl[])
                          }
                          frame "milliAmps".. {
                            # "Converts nA to mA"
                            n248 = Divide(x=w458, y=1000000.0) -> (x/y=w456:dbl[])
                          }
                        }
                        n249 = property on="Igraph" class="XYGraph (strict)"("YScale.Minimum"=w409) -> ()  [unwired: 2 in, 2 out]
                        n250 = for {
                          N: 4 -> [_]
                          tunnel: w416 -> [w432]
                          tunnel: w414 -> [w431]
                          tunnel: w408 -> [w428]
                          i -> [w433]
                          # "Update \"Last 5 readings:\" IV indicator and T/RH indicators"
                          n251 = call "IVData.vi"("Action"=T3."Read Array", "Array No."=w433) -> ("Array OUT"=w430:dbl[])  [unwired: 3 in, 1 out]
                          n252 = case shown="..0" w433 {
                            tunnel: w432 -> [w436 w440 _ _]
                            tunnel: w431 -> [w437 w441 _ _]
                            tunnel: w430 -> [w435 w439 w445 w450]
                            tunnel: w428 -> [_ _ w443 w448]
                            frame ..0 {
                              # "Read Voltage from 1st column"
                              n253 = Array Subset(array=w435, index=w437, length=w436) -> (w434:dbl[])
                              n254 = local write "Volts"(w434) -> ()
                            }
                            frame 1 {
                              # "Read Current from 2nd column"
                              n255 = Array Subset(array=w439, index=w441, length=w440) -> (w438:dbl[])
                              n256 = local write "Current"(w438) -> ()
                            }
                            frame 2 {
                              # "Read Temperature from 3rd column"
                              n257 = Decrement(x=w443) -> (x-1=w442:u32)
                              n258 = Array Subset(array=w445, index=w442, length=1) -> (w444:dbl[])
                              n259 = local write "Temp."(w444) -> ()
                            }
                            frame 3.. {
                              # "Read Relative Humidity from 4th column"
                              n260 = Decrement(x=w448) -> (x-1=w447:u32)
                              n261 = Array Subset(array=w450, index=w447, length=1) -> (w449:dbl[])
                              n262 = local write "RH"(w449) -> ()
                            }
                          }
                        }
                        n263 = Bundle(w399, w422) -> (w410:cluster{dbl[], dbl[]})  [unwired: 1 in]
                        n264 = local write "Igraph"(w410) -> ()
                      }
                      frame #2 {
                        # "Increase volts and check for end of ramp"
                        # "Increase voltage and check compliance"
                        n265 = local read "Current Volts:"() -> (w462:dbl)
                        n266 = local read "Current Volts:"() -> (w459:dbl)
                        n267 = local read "positive ramp?"() -> (w471:bool)
                        n268 = Quotient & Remainder(x=w459, y=w467) -> (x-y*floor(x/y)=w468:dbl, floor(x/y)=w466:dbl)
                        n269 = case shown="False" w471 {
                          tunnel: w467 -> [w478 w482]
                          tunnel: w475 -> [w479 w485]
                          tunnel: [w477 w484] -> w463
                          tunnel: [w476 w481] -> w474
                          tunnel: w462 -> [w480 w483]
                          frame False {
                            n270 = Subtract(x=w480, y=w479) -> (x-y=w476:dbl)
                            n271 = Greater Or Equal?(x=w476, y=w478) -> (x >= y?=w477:bool)
                          }
                          frame True {
                            n272 = Add(x=w483, y=w485) -> (x+y=w481:dbl)
                            n273 = Less Or Equal?(x=w481, y=w482) -> (x <= y?=w484:bool)
                          }
                        }
                        n274 = Not Equal To 0?(x=w468) -> (x != 0?=w464:bool)
                        n275 = Equal To 0?(x=w466) -> (x = 0?=w465:bool)
                        n276 = Or(x=w464, y=w465) -> ()  [unwired: 1 out]
                        n277 = case shown="False" w463 {
                          tunnel: w474 -> [_ w501]
                          tunnel: [w489 FALSE] -> w473
                          tunnel: [FALSE w491] -> w472
                          tunnel: w459 -> [_ w499]
                          tunnel: w470 -> [_ w498]
                          tunnel: w469 -> [_ w497]
                          tunnel: w461 -> [w488 _]
                          tunnel: [w487 0] -> w460
                          frame False {
                            (unwired) TRUE
                            n278 = Increment(x=w488) -> (x+1=w487:i32)
                            n279 = local read "hold steps"() -> (w486:i32)
                            n280 = Greater Or Equal?(x=w488, y=w486) -> (x >= y?=w489:bool)
                          }
                          frame True {
                            # "Message \"Incrementing volts.\""
                            # "Increase  voltage, check compliance and check PTP supply errors"
                            n281 = local read "step [V]"() -> (w495:dbl)
                            n282 = call "SupplyRamp.vi"("error in"=w498, "Requested Voltage"=w501, "Step Size"=w495, "Step Delay"=100, "Supply IN"=w497, "Starting Voltage"=w499) -> ("error out"=w493:errorcluster, "Compliance exceeded"=w491:bool, "Current Voltage"=w496:dbl)  [unwired: 2 in, 1 out]
                            n283 = local write "STATUS 1"("Incrementing volts.") -> ()
                            n284 = case shown="No Error" w493 {
                              tunnel: w496 -> [w503 _]
                              frame No Error {
                                n285 = local write "Current Volts:"(w503) -> ()
                              }
                              frame Error {
                              }
                            }
                            n286 = property on="Bias On/Off:" class="Bool (strict)"("Blinking"=w491) -> ()  [unwired: 2 in, 2 out]
                          }
                        }
                      }
                    }
                  }
                  frame True {
                    w505 = FALSE
                    # "\"ABORT\" button pressed"
                  }
                }
              }
            }
            n287 = case shown="False" w255 {
              frame False {
              }
              frame True {
                n288 = property on="Bias On/Off:" class="Bool (strict)"("Blinking"=TRUE) -> ()  [unwired: 2 in, 2 out]
              }
            }
            n289 = Build Array(w256, w255, "abort", w251) -> (w260:bool[])
            n290 = Or Array Elements(Boolean array=w260) -> (logical OR=w266:bool)
            n291 = Not(x=w266) -> (.not. x?=w265:bool)
          }
        }
        frame True {
          w507 = FALSE
          # "Flag compliance as reason for end of run"
          # "Compliance exceeded when first voltage applied"
          n292 = local write "STATUS 1"("Run aborted - compliance exceeded.") -> ()
          n293 = Build Array(w507, TRUE, w507, w507) -> (w508:bool[])
        }
      }
      n294 = Search 1D Array(1D array=w240, element=TRUE) -> (index of element=w238:i32)  [unwired: 1 in]
      n295 = Increment(x=w238) -> (x+1=w237:i32)
      n296 = case shown="1" w237 {
        tunnel: ["" "Run ended normally" "Compliance exceeded" "Run aborted - by user" "Run aborted - Ilimit exceeded"] -> w232
        frame ..0 {
        }
        frame 1 {
        }
        frame 2 {
        }
        frame 3 {
        }
        frame 4.. {
        }
      }
      n297 = Concatenate Strings(w232, "\r\n", "RAMPING DOWN VOLTS") -> (w235:string)
      n298 = global read "QC_RunInformation.vi" "Run info"() -> (w236:T7)
      n299 = Bundle By Name(cluster=w236, "End of Run comment:"=w232) -> (w231:T7)
      n300 = local write "STATUS 1"(w235) -> ()
      n301 = global write "QC_RunInformation.vi" "Run info"(w231) -> ()
    }
    frame #4 {
      # "Ramp down, switch off supply, ask to save data and save jpg of the Front Panel"
      n302 = stacked-sequence {
        frame #0 {
          # "Switch IV supply to STANDBY"
          # "s -> ms"
          # "Ramp down voltage and switch IV supply to standby"
          n303 = global read "QC_MeasurementSetup.vi" "IV Measurement Parameters"() -> (w519:T6)
          n304 = Unbundle By Name(w519) -> ("Supply"=w518:refnum<class "SupplyControl.lvclass">, "Ramp down Interval [s]"=w511:i32, "Ramp down steps [V]"=w512:dbl, "Switching"=w513:refnum<class "Switching.lvclass">, "Matrix used?"=w514:bool)
          n305 = local read "Current Volts:"() -> (w524:dbl)
          n306 = Multiply(x=w511, y=1000) -> (x*y=w521:i32)
          n307 = call "SupplyRamp.vi"("Requested Voltage"=0.0, "Step Size"=w512, "Step Delay"=w521, "Supply IN"=w518, "Starting Voltage"=w524) -> ("error out"=w517:errorcluster, "Supply OUT"=w516:refnum<class "SupplyControl.lvclass">, "Current Voltage"=w522:dbl)  [unwired: 3 in, 1 out]
          n308 = local write "Current Volts:"(w522) -> ()
          n309 = call-dynamic "Supply_Stby.vi"("error in (no error)"=w517, "SupplyControl in"=w516) -> ("error out"=w515:errorcluster)  [unwired: 8 in, 1 out]
          n310 = case shown="True" w514 {
            tunnel: w513 -> [_ w529]
            tunnel: w515 -> [_ w528]
            frame False {
            }
            frame True {
              # "CLOSE Switching Matrix"
              # "RESET Switching  Matrix"
              n311 = call-dynamic "MatrixSwitch.vi"("error in (no error)"=w528, "Action"=T4."Reset", "Switching in"=w529) -> ("error out"=w525:errorcluster, "Switching out"=w526:refnum<class "Switching.lvclass">)  [unwired: 6 in, 1 out]
              n312 = call-dynamic "Close.vi"("error in (no error)"=w525, "Switching in"=w526) -> ()  [unwired: 8 in, 2 out]
            }
          }
        }
        frame #1 {
          w534 = 0
          # "\"Current Volts\" indicator back to 0.00 V"
          # "\"Bias  On/Off\" indicator in Off (red)"
          # "\"ABORT\" button disanabled \nand dimmed (Disabled=2)"
          # "\"QUIT\" and \"Save & QUIT\" buttons \nenabled (Disabled=0)"
          # "Reset \"Current Volts\" and \"Bias On/Off\" indicators, \"ABORT\" button disabled and \"QUIT\"/\"Save & QUIT\" buttons enabled"
          n313 = property on="Quit & Save" class="Bool"("DisabledEnum"=w534) -> ()  [unwired: 2 in, 2 out]
          n314 = property on="quit (no save)" class="Bool"("DisabledEnum"=w534) -> ()  [unwired: 2 in, 2 out]
          n315 = local write "Current Volts:"(0.0 ("Current Volts:")) -> ()
          n316 = property on="abort" class="Bool (strict)"("DisabledEnum"=2) -> ()  [unwired: 2 in, 2 out]
          n317 = local write "Bias On/Off:"(FALSE ("Visible")) -> ()
          n318 = local write "STATUS 1"("Run finished. \nSave data?" ("STATUS 1")) -> ()
        }
        frame #2 {
          # "Save  jpg  image of the Front Panel"
          n319 = Current VI's Path() -> (path=w536:path)
          n320 = call "SaveJPEG.vi"("Test"="IV", "File Path Control"=w536) -> ()  [unwired: 1 in, 2 out]
        }
      }
    }
    frame #5 {
      # "*WARNING*: \"Done!\" indicator in \nFront Panel hidden."
      # "Switch off Arduino if used for T/RH measurement"
      # "Display and save data"
      n321 = local read "Scales"() -> (w547:T1)
      n322 = global read "QC_MeasurementSetup.vi" "IV Measurement Parameters"() -> (w545:T6)
      n323 = local read "Iscale"() -> (w546:enum16{"nanoAmps", "microAmps", "milliAmps"})
      n324 = while {
        shift-left: w546 -> [w592]
        shift-right: [w591] -> _
        shift-left: w547 -> [w594]
        shift-right: [w593] -> _
        tunnel: ["Quit & Save"] -> w549
        tunnel: ["quit (no save)"] -> w548
        stop <- w589 continue-if-true
        # "Loop and await decision on whether to save or junk data"
        n325 = local read "Scales"() -> (w593:T1)
        n326 = local read "Iscale"() -> (w591:enum16{"nanoAmps", "microAmps", "milliAmps"})
        n327 = Not Equal?(x=w594, y=w593) -> (x != y?=w587:bool)
        n328 = Not Equal?(x=w592, y=w591) -> (x != y?=w586:bool)
        n329 = case shown="True" w587 {
          tunnel: w593 -> [_ w621]
          frame False {
          }
          frame True {
            # "Allow to change the IV plot representation (Linear=0, Logarithmic=1)"
            n330 = case shown="..\"Lin - Lin\"" w621 {
              tunnel: [w622 1 0 w627] -> w620
              tunnel: [w622 0 1 w627] -> w619
              frame .."Lin - Lin" {
                w622 = 0
              }
              frame "Log - Lin" {
              }
              frame "Lin - Log" {
              }
              frame "Log - log".. {
                w627 = 1
              }
            }
            n331 = property on="Igraph" class="XYGraph (strict)"("X Scale.Mapping Mode"=w620) -> ()  [unwired: 2 in, 2 out]
            n332 = property on="Igraph" class="XYGraph (strict)"("Y Scale.Mapping Mode"=w619, "YScale.Minimum"=w619) -> ()  [unwired: 2 in, 2 out]
          }
        }
        n333 = case shown="True" w586 {
          tunnel: w591 -> [_ w607]
          frame False {
          }
          frame True {
            w600 = T3."Read Array" ("Action")
            # "Set minimum in Current (Y) axis in 0 if linear and 1 if logarithmic"
            # "Allow to change the Current scale (nA, µA or mA)"
            n334 = global read "QC_MeasurementSetup.vi" "IV Measurement Parameters"() -> (w602:T6)
            n335 = property on="Igraph" class="XYGraph (strict)"() -> ("YScale.Mapping Mode"=w603:u8)  [unwired: 2 in, 2 out]
            n336 = property on="Igraph" class="XYGraph (strict)"("YScale.Minimum"=w603) -> ()  [unwired: 2 in, 2 out]
            n337 = Unbundle By Name(w602) -> ("Number Of Steps"=w599:u32)
            n338 = local read "hold steps"() -> (w598:i32)
            n339 = Add(x=w599, y=w598) -> (x+y=w597:u32)
            n340 = call "IVData.vi"("Action"=w600, "Array No."=u32 1 ("Action")) -> ("Array OUT"=w609:dbl[])  [unwired: 3 in, 1 out]
            n341 = Array Subset(array=w609, index=0, length=w597) -> (w606:dbl[])
            n342 = Absolute Value(x=w606) -> (abs(x)=w605:dbl[])
            n343 = call "IVData.vi"("Action"=w600, "Array No."=u32 0 ("Action")) -> ("Array OUT"=w596:dbl[])  [unwired: 3 in, 1 out]
            n344 = case shown="\"microAmps\"" w607 {
              tunnel: [w612 w613 w617] -> w611
              tunnel: w605 -> [w612 w615 w618]
              frame .."nanoAmps" {
              }
              frame "microAmps" {
                n345 = Divide(x=w615, y=1000.0) -> (x/y=w613:dbl[])
              }
              frame "milliAmps".. {
                n346 = Divide(x=w618, y=1000000.0) -> (x/y=w617:dbl[])
              }
            }
            n347 = Absolute Value(x=w596) -> (abs(x)=w595:dbl[])
            n348 = Bundle(w595, w611) -> (w608:cluster{dbl[], dbl[]})  [unwired: 1 in]
            n349 = local write "Igraph"(w608) -> ()
          }
        }
        n350 = Not Or(1:"quit (no save)", 2:"Quit & Save") -> (0:w589:bool)
      }
      n351 = Unbundle By Name(w545) -> ("Temperature Readout"=w544:enum16{"Read Arduino", "Enter manually"}, "Arduino"=w538:refnum<class "ArduinoControl.lvclass">)
      n352 = case shown="\"Read Arduino\"" w544 {
        tunnel: w538 -> [_ w585]
        frame "Enter manually", Default {
        }
        frame "Read Arduino" {
          n353 = call "ArduinoClose.vi"("ArduinoControl in"=w585) -> ()  [unwired: 9 in, 2 out]
        }
      }
      n354 = case shown="True" w548 {
        tunnel: [FALSE w629] -> w550
        frame False {
        }
        frame True {
          n355 = Two Button Dialog(message="Are you sure you don't want to save the data?", 1:"Quit" ("F button name (\"Cancel\")"), 2:"Save data" ("T button name (\"OK\")")) -> (T button?=w629:bool)
        }
      }
      n356 = Or(x=w549, y=w550) -> (x .or. y?=w543:bool)
      n357 = flat-sequence {
        tunnel: w543 -> [w553]
        tunnel: [w553] -> w539
        tunnel: [TRUE] -> w537
        frame #0 {
          # "Extract breakdown voltage"
          n358 = global read "QC_MeasurementSetup.vi" "IV Measurement Parameters"() -> (w562:T6)
          n359 = Unbundle By Name(w562) -> ("V_breakdown Limit [V]"=w556:dbl, "Number Of Steps"=w557:u32)
          n360 = call "ScanFeedback.vi"("measurement type"=T5."IV") -> ("V breakdown"=w551:dbl)  [unwired: 4 in, 4 out]
          n361 = Absolute Value(x=w551) -> (abs(x)=w554:dbl)
          n362 = Absolute Value(x=w556) -> (abs(x)=w555:dbl)
          n363 = Greater Or Equal?(x=w554, y=w555) -> (x >= y?=w558:bool)
          n364 = case shown="True" w553 {
            tunnel: ["" w584] -> w563
            tunnel: [_ w569] -> w561
            tunnel: w557 -> [_ w567]
            frame False {
            }
            frame True {
              w580 = T3."Read Array" ("Action")
              # "Show \"Saving Data ...\" message"
              # "Save data in file"
              n365 = local read "hold steps"() -> (w566:i32)
              n366 = local write "STATUS 1"("Saving Data ...") -> ()
              n367 = Add(x=w567, y=w566) -> ()  [unwired: 1 out]
              n368 = call "IVData.vi"("Action"=w580, "Array No."=u32 0 ("Action")) -> ("Array OUT"=w575:dbl[])  [unwired: 3 in, 1 out]
              n369 = call "IVData.vi"("Action"=w580, "Array No."=u32 1 ("Action")) -> ("Array OUT"=w574:dbl[])  [unwired: 3 in, 1 out]
              n370 = Build Array(w575, w574) -> (w573:dbl[][])
              n371 = Transpose 2D Array(2D array=w573) -> (transposed array=w572:dbl[][])
              n372 = call "IVData.vi"("Action"=w580, "Array No."=u32 2 ("Action")) -> ("Array OUT"=w582:dbl[])  [unwired: 3 in, 1 out]
              n373 = call "IVData.vi"("Action"=w580, "Array No."=u32 3 ("Action")) -> ("Array OUT"=w581:dbl[])  [unwired: 3 in, 1 out]
              n374 = call <vilib>:"Std Deviation and Variance.vi"("X"=w582) -> ("mean"=w570:dbl)  [unwired: 1 in, 2 out]
              n375 = call <vilib>:"Std Deviation and Variance.vi"("X"=w581) -> ("mean"=w571:dbl)  [unwired: 1 in, 2 out]
              n376 = call "SaveDataFile.vi"("Data Array"=w572, "Temperature"=w571, "Humidity"=w570, "Array Titles"="Voltage[V] Current[nA]", "Strip Segment"="") -> ("Path + Filename OUT"=w584:string, "Error Out"=w569:errorcluster)  [unwired: 7 in, 2 out]
            }
          }
          n377 = call "WriteLogFile.vi"("Automatic warning"="", "Data File"=w563, "Error In"=w561, "DUT passed?"=w558, "Value TechSpec criteria"=w551, "Files saved?"=w553) -> ()  [unwired: 5 in, 1 out]
        }
      }
      n378 = Select(t="Run finished.\nData saved." ("STATUS 1"), s=w539, f="Run finished.\nData not saved." ("STATUS 1")) -> (s? t:f=w542:string)
      n379 = local write "STATUS 1"(w542) -> ()
      "Done!" <- w537
    }
  }
